vi "TSPopup.Init Controls.vi"(9 "Font Size":u32, 11 "Popup Cluster Ref":refnum<vi>) -> (3 "dup ref":refnum<vi>, 5 "Offsets":cluster{"Left":i32, "Top":i32}[](array[cluster]))   [LabVIEW 2013]
doc: "Initializes the popup cluster and its controls.\n\nType Sensitive Popup \nCopyright © 2007, J. David Saunders\nAll rights reserved."
panel:
  # "Type Sensitive Popup \nCopyright © 2007, J. David Saunders\nAll rights reserved."
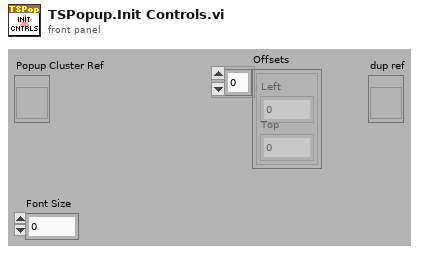
[diagram p1: front panel]
types:
  T1 = typedef "LVPositionTypeDef.ctl" = cluster{"Left":i32, "Top":i32}
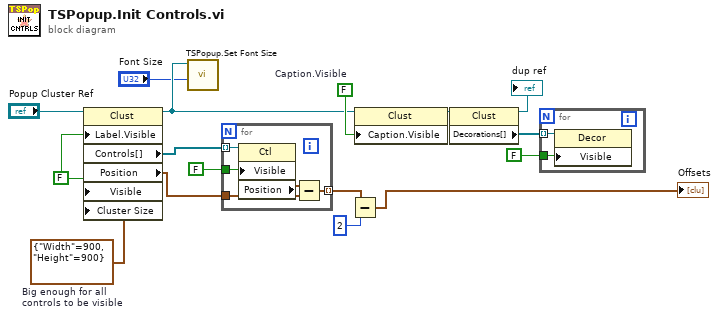
[diagram p0: block diagram]
diagram:
  w4 = FALSE  # Caption.Visible
  w12 = cluster{"Width":u32, "Height":u32} {"Width"=900, "Height"=900}  # Big enough for all controls to be visible
  w13 = FALSE ("Wait until done")
  n1 = property class="Clust"(reference="Popup Cluster Ref", "Label.Visible"=w13, "Visible"=w13, "Cluster Size"=w12) -> (reference out=w2:refnum<vi>, "Controls[]"=w3:refnum<vi>[], "Position"=w7:T1)  [unwired: 1 in, 1 out]
  n2 = call "TSPopup.Set Font Size.vi"("Font Size"="Font Size", "Popup Cluster Ref"=w2) -> ()  [unwired: 8 in, 2 out]
  n3 = for {
    tunnel: w3 -> [w21] mode=indexing
    tunnel: w7 -> [w19]
    tunnel: [w18] -> w14 mode=indexing
    tunnel: FALSE ("Wait until done") -> [w17]
    n4 = property class="Ctl"(reference=w21, "Visible"=w17) -> ("Position"=w20:T1)  [unwired: 1 in, 2 out]
    n5 = Subtract(x=w20, y=w19) -> (x-y=w18:T1)
  }
  n6 = Subtract(x=w14, y=2) -> (x-y=→"Offsets":T1[])
  n7 = property class="Clust"(reference=w2, "Caption.Visible"=w4) -> (reference out=w5:refnum<vi>)  [unwired: 1 in, 1 out]
  n8 = property class="Clust"(reference=w5) -> (reference out=→"dup ref":refnum<vi>, "Decorations[]"=w10:refnum<vi>[])  [unwired: 1 in, 1 out]
  n9 = for {
    tunnel: w10 -> [w23] mode=indexing
    tunnel: FALSE ("Visible") -> [w22]
    n10 = property class="Decor"(reference=w23, "Visible"=w22) -> ()  [unwired: 1 in, 2 out]
  }
